vi "ReadActiveConfiguration.vi"(8 "error in (no error)":errorcluster, 11 "VeriStandTestCase in":refnum<class "VeriStandTestCase.lvclass">) -> (0 "error out":errorcluster, 2 "Target Platform":T1, 3 "VeriStandTestCase out":refnum<class "VeriStandTestCase.lvclass">)   [LabVIEW 2027, in "VeriStandTestCase.lvclass"]
uses:
  VeriStandTestCase.lvclass
  VeriStandTestUtilities/TargetPlatform.ctl
  VeriStandTestCase.lvclass/VeriStandTestCase.ctl
  VeriStandTestUtilities/VeriStandTestUtilities.lvlib
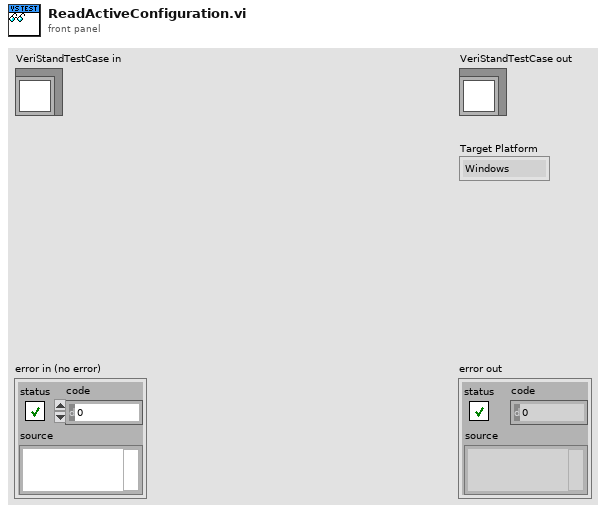
[diagram p1: front panel]
types:
  T1 = typedef "VeriStandTestUtilities.lvlib/TargetPlatform.ctl" = enum16{"Windows", "Linux64CRIO", "Linux64PXI", "LinuxARM", "PharLap"}
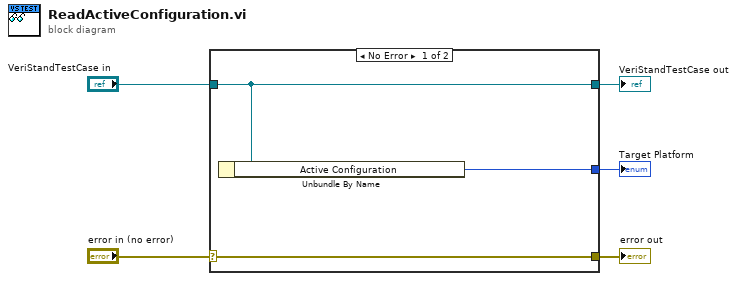
[diagram p0: block diagram]
diagram:
  n1 = case shown="No Error" "error in (no error)" {
    selector: "error in (no error)" -> [w8 w9]
    tunnel: [w8 w9] -> w4
    tunnel: [w7 w10] -> w2
    tunnel: "VeriStandTestCase in" -> [w7 w10]
    tunnel: [w6 _] -> w1
    frame No Error {
      n2 = Unbundle By Name(w7) -> ("Active Configuration"=w6:T1)
    }
    frame Error {
    }
  }
  "error out" <- w4
  "VeriStandTestCase out" <- w2
  "Target Platform" <- w1
